vi "WPI_CANTalonSRX_ScaleUnits.vi"(5 "Feedback Scalar Select":T1 items=["Digital Quadrature Encoder"=0, "Analog Pot"=2, "Analog Encoder"=3, "Count on Quad-A (Rising-Edge)"=4, "Count on Quad-A (Falling-Edge)"=5, "Position is Pulse-Width"=8, "CTR Magnetic Enc (Relative)"=6, "CTR Magnetic Enc (Absolute)"=7], 7 "Read For Send":T2={"Output"=0.0, "Control Mode"=enum."Percent VBus", "Brake-Mode Override"=enum."No Override", "Reverse Feedback Sensor"=FALSE, "Reverse Closed-Loop Output"=FALSE, "Override Limits"=FALSE, "Forward Limit Enabled"=FALSE, "Reverse Limit Enabled"=FALSE, "Feedback Select"=0, "Profile Select"=0, "Master To Follow"=0, "Throttle Ramp Rate"=0, "Disabled"=FALSE, "Encoder Codes Per Rev"=0, "Num Pot Turns"=0, "Control Frame Rate Ms"=0, "Use Control5 If Supported"=TRUE, "Enable Frame Rate Ms"=10, "Motion Profile Flow Control"=0, "Motion Profile Control Frame Rate"=10, "Talon SRX Motion Profile Trajectory Point"={"Duration Ms"=0, "Velocity"=0.0, "Position"=0.0, "Profile Slot Select"=0, "Is Last"=FALSE, "Velocity Only"=FALSE, "Zero Position"=FALSE, "Compress Code"=0, "Same Velocity"=0, "Delta Position"=0, "Count"=0}, "Current Limit Enabled"=FALSE} {"Feedback Select" items=["Digital Quadrature Encoder"=0, "Analog Pot"=2, "Analog Encoder"=3, "Count on Quad-A (Rising-Edge)"=4, "Count on Quad-A (Falling-Edge)"=5, "Position is Pulse-Width"=8, "CTR Magnetic Enc (Relative)"=6, "CTR Magnetic Enc (Absolute)"=7]}) -> (4 "Position Scalar":dbl, 8 "Velocity Scalar":dbl, 15 "Scalar Is Valid":bool)   [LabVIEW 2016]
uses:
  WPI_CANTalonSRX_GlobalControl.ctl
  WPI_CANTalonSRX_APIControlMode.ctl
  WPI_CANTalonSRX_BrakeOverride.ctl
  WPI_CANTalonSRX_FeedbackSelect.ctl
  WPI_CANTalonSRX_MotionProfileTrajectoryPt.ctl
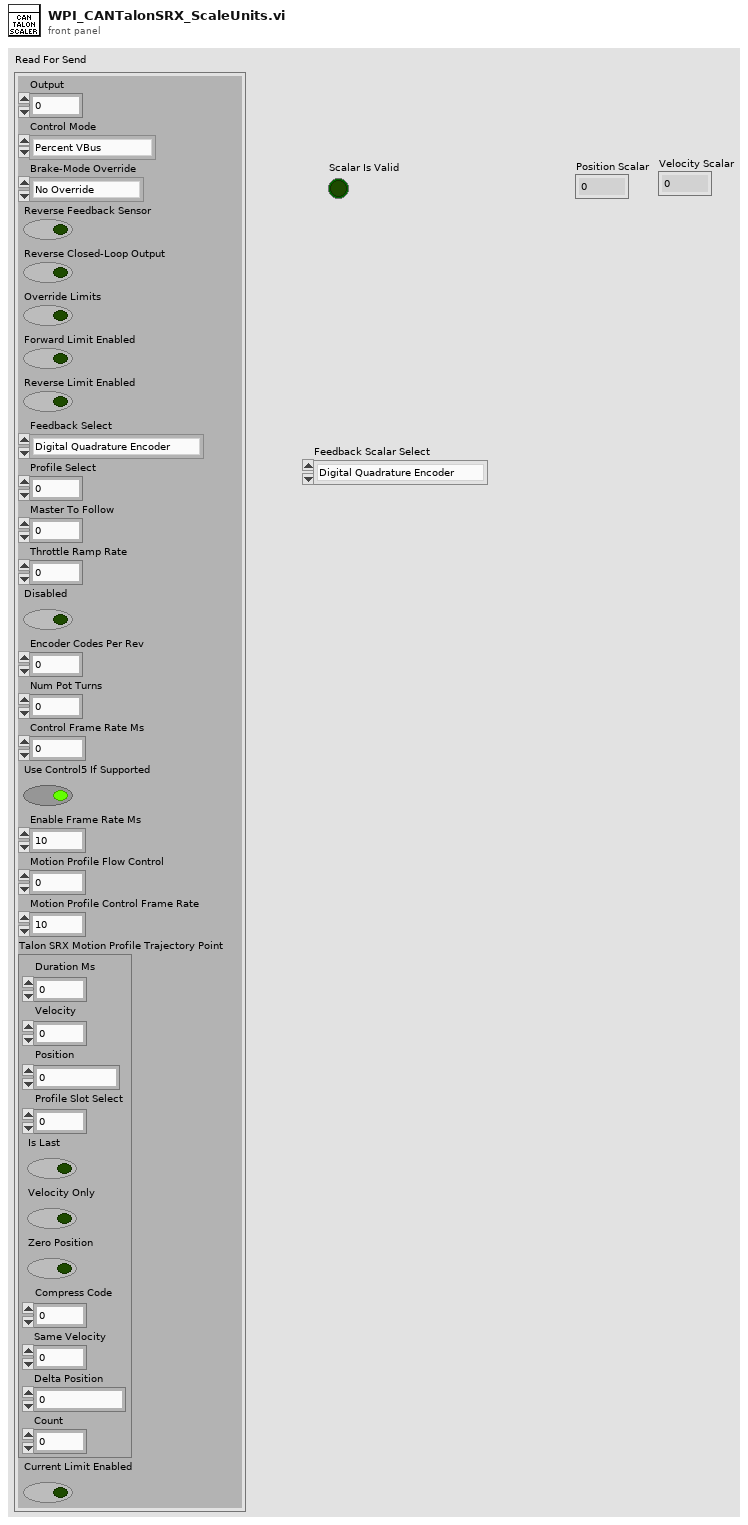
[diagram p1: front panel]
types:
  T1 = typedef "WPI_CANTalonSRX_FeedbackSelect.ctl" = u8
  T2 = typedef "WPI_CANTalonSRX_GlobalControl.ctl" = cluster{"Output":dbl, "Control Mode":T3, "Brake-Mode Override":T4, "Reverse Feedback Sensor":bool, "Reverse Closed-Loop Output":bool, "Override Limits":bool, "Forward Limit Enabled":bool, "Reverse Limit Enabled":bool, "Feedback Select":T1, "Profile Select":u8, "Master To Follow":u8, "Throttle Ramp Rate":u8, "Disabled":bool, "Encoder Codes Per Rev":u32, "Num Pot Turns":u32, "Control Frame Rate Ms":u8, "Use Control5 If Supported":bool, "Enable Frame Rate Ms":u8, "Motion Profile Flow Control":u8, "Motion Profile Control Frame Rate":u8, "Talon SRX Motion Profile Trajectory Point":T5, "Current Limit Enabled":bool}
  T3 = typedef "WPI_CANTalonSRX_APIControlMode.ctl" = enum8{"Percent VBus", "Speed", "Position", "Slave", "Unchanged / Invalid", "Voltage Compensation", "Current", "Motion Profile", "Motion Magic"}
  T4 = typedef "WPI_CANTalonSRX_BrakeOverride.ctl" = enum8{"No Override", "Override to Coast", "Override to Brake"}
  T5 = typedef "WPI_CANTalonSRX_MotionProfileTrajectoryPt.ctl" = cluster{"Duration Ms":u8, "Velocity":dbl, "Position":dbl, "Profile Slot Select":u8, "Is Last":bool, "Velocity Only":bool, "Zero Position":bool, "Compress Code":u8, "Same Velocity":i32, "Delta Position":i32, "Count":u8}
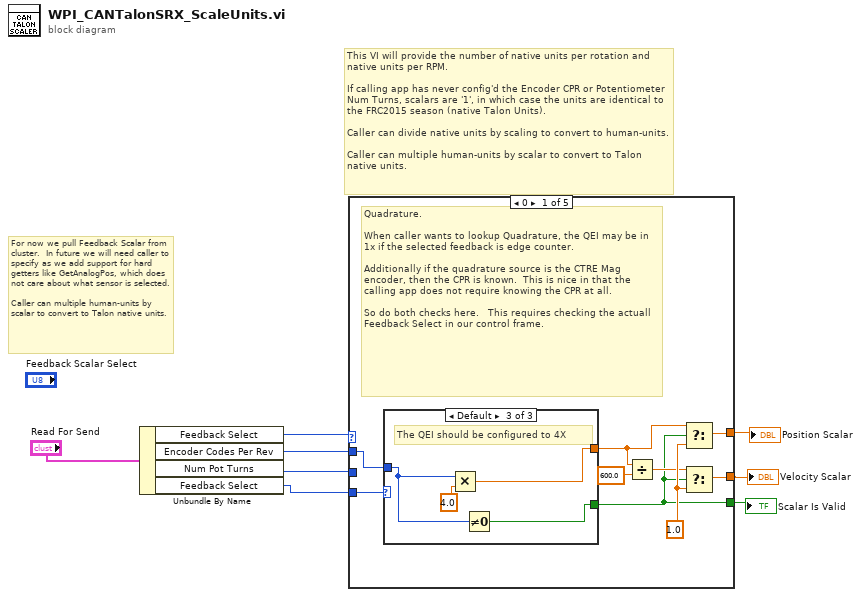
[diagram p0: block diagram]
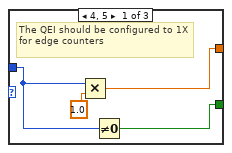
[diagram p2: hidden frame]
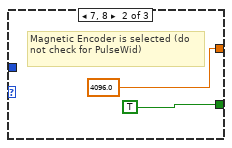
[diagram p3: hidden frame]
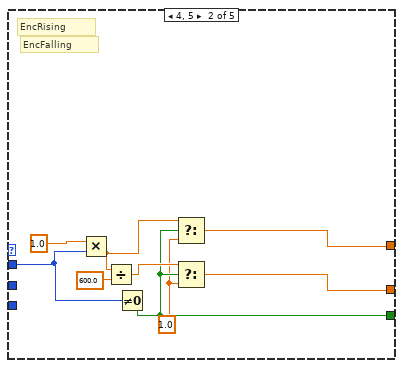
[diagram p4: hidden frame]
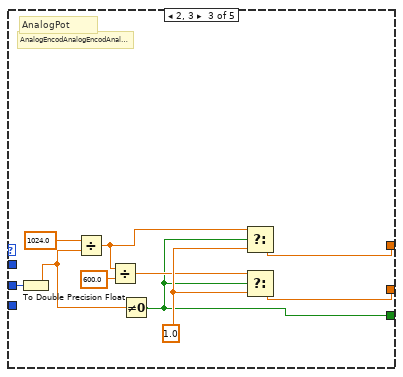
[diagram p5: hidden frame]
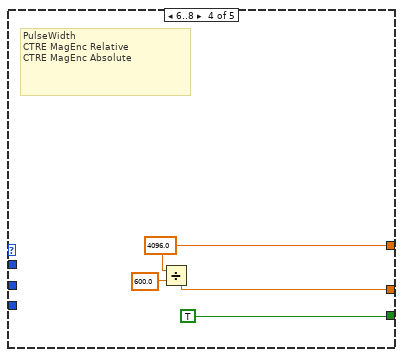
[diagram p6: hidden frame]
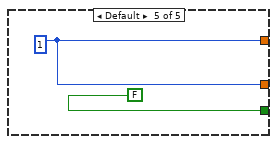
[diagram p7: hidden frame]
diagram:
  # "For now we pull Feedback Scalar from cluster.  In future we will need caller to specify as we add support for hard getters like GetAnalogPos, which does not care about what sensor is selected.\n\nCaller can multiple human-units by scalar to convert to Talon native units."
  # "This VI will provide the number of native units per rotation and native units per RPM.\n\nIf calling app has never config'd the Encoder CPR or Potentiometer Num Turns, scalars are '1', in which case the units are identical to the FRC2015 season (native Talon Units).\n\nCaller can divide native units by scaling to convert to human-units.\n\nCaller can multiple human-units by scalar to convert to Talon native units."
  n1 = Unbundle By Name("Read For Send") -> ("Feedback Select"=w1:T1, "Encoder Codes Per Rev"=w4:u32, "Num Pot Turns"=w5:u32, "Feedback Select"=w2:T1)
  n2 = case shown="0" w1 {
    tunnel: [w12 w33 w37 w48 w52] -> w8
    tunnel: [w11 w29 w38 w49 w52] -> w6
    tunnel: w4 -> [w9 w34 _ _ _]
    tunnel: [w13 w30 w39 TRUE ("Scalar Is Valid") FALSE ("Scalar Is Valid")] -> w7
    tunnel: w5 -> [_ _ w44 _ _]
    tunnel: w2 -> [w10 _ _ _ _]
    frame 0 {
      w16 = 1.0 ("y")
      # "Quadrature.      \n\nWhen caller wants to lookup Quadrature, the QEI may be in 1x if the selected feedback is edge counter.  \n\nAdditionally if the quadrature source is the CTRE Mag encoder, then the CPR is known.  This is nice in that the calling app does not require knowing the CPR at all.\n\nSo do both checks here.   This requires checking the actuall Feedback Select in our control frame."
      n3 = case shown="Default" w10 {
        tunnel: w9 -> [w20 _ w24]
        tunnel: [w19 4096.0 ("y") w27] -> w14
        tunnel: [w18 TRUE w26] -> w13
        frame 4, 5 {
          # "The QEI should be configured to 1X for edge counters"
          n4 = Multiply(x=w20, y=1.0) -> (x*y=w19:dbl)
          n5 = Not Equal To 0?(x=w20) -> (x != 0?=w18:bool)
        }
        frame 7, 8 {
          # "Magnetic Encoder is selected (do not check for PulseWid)"
        }
        frame Default {
          # "The QEI should be configured to 4X"
          n6 = Multiply(x=w24, y=4.0) -> (x*y=w27:dbl)
          n7 = Not Equal To 0?(x=w24) -> (x != 0?=w26:bool)
        }
      }
      n8 = Divide(x=w14, y=600.0) -> (x/y=w15:dbl)
      n9 = Select(t=w14, s=w13, f=w16) -> (s? t:f=w12:dbl)
      n10 = Select(t=w15, s=w13, f=w16) -> (s? t:f=w11:dbl)
    }
    frame 4, 5 {
      w28 = 1.0 ("y")
      # "EncFalling"
      # "EncRising"
      n11 = Multiply(x=1.0 ("y"), y=w34) -> (x*y=w31:dbl)
      n12 = Divide(x=w31, y=600.0) -> (x/y=w32:dbl)
      n13 = Not Equal To 0?(x=w34) -> (x != 0?=w30:bool)
      n14 = Select(t=w31, s=w30, f=w28) -> (s? t:f=w33:dbl)
      n15 = Select(t=w32, s=w30, f=w28) -> (s? t:f=w29:dbl)
    }
    frame 2, 3 {
      w42 = 1.0 ("y")
      # "AnalogEncodAnalogEncodAnalogEncoder"
      # "AnalogPot"
      n16 = To Double Precision Float(number=w44) -> (double precision float=w43:dbl)
      n17 = Divide(x=1024.0 ("y"), y=w43) -> (x/y=w41:dbl)
      n18 = Divide(x=w41, y=600.0) -> (x/y=w40:dbl)
      n19 = Not Equal To 0?(x=w43) -> (x != 0?=w39:bool)
      n20 = Select(t=w41, s=w39, f=w42) -> (s? t:f=w37:dbl)
      n21 = Select(t=w40, s=w39, f=w42) -> (s? t:f=w38:dbl)
    }
    frame 6..8 {
      w48 = 4096.0 ("y")
      # "PulseWidth\nCTRE MagEnc Relative \nCTRE MagEnc Absolute"
      n22 = Divide(x=w48, y=600.0) -> (x/y=w49:dbl)
    }
    frame Default {
      w52 = u8 1 ("Device ID (0)")
    }
  }
  "Position Scalar" <- w8
  "Velocity Scalar" <- w6
  "Scalar Is Valid" <- w7
